vi "Init UART.vi"(6 "Term Char":string, 8 "error in (no error)":errorcluster, 9 "Baud":u32=115200, 10 "UART In":T1=-1, 11 "Session in":refnum<class "Session.lvclass">) -> (0 "error out":errorcluster, 3 "Session out":refnum<class "Session.lvclass">)   [LabVIEW 2020, in "CTI.lvlib" / "Session.lvclass"]
uses:
  Session.lvclass
  Session.lvclass/Session.ctl
  UART/UART.lvclass
  DeviceComms/DeviceComms.lvclass
  UART Number.ctl
  CTI.lvlib
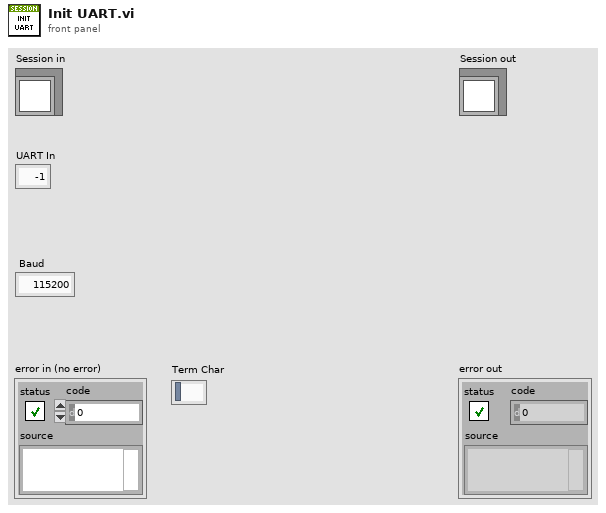
[diagram p1: front panel]
types:
  T1 = typedef "CTI.lvlib/UART Number.ctl" = i8
  T2 = typedef "CTI.lvlib/GPIO Number.ctl" = i8
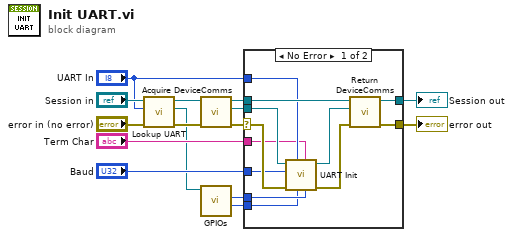
[diagram p0: block diagram]
diagram:
  n1 = call "Lookup UART.vi"("error in (no error)"="error in (no error)", "UART #"="UART In", "Session in"="Session in") -> ("error out"=w5:errorcluster, "UART"=w1:refnum<class "UART.lvclass">, "Session out"=w3:refnum<class "Session.lvclass">)  [unwired: 6 in]
  n2 = call "Acquire DeviceComms.vi"("error in (no error)"=w5, "Session in"=w3) -> ("error out"=w6:errorcluster, "DeviceComms"=w11:refnum<class "DeviceComms.lvclass">, "Session out"=w13:refnum<class "Session.lvclass">)  [unwired: 7 in]
  n3 = call "GPIOs.vi"("UART in"=w1) -> ("RX GPIO"=w7:T2, "TX GPIO"=w8:T2)  [unwired: 7 in, 2 out]
  n4 = case shown="No Error" w6 {
    selector: w6 -> [w27 w29]
    tunnel: [w26 w29] -> w14
    tunnel: w13 -> [w25 w28]
    tunnel: [w24 w28] -> w12
    tunnel: w11 -> [w23 _]
    tunnel: "UART In" -> [w22 _]
    tunnel: "Term Char" -> [w21 _]
    tunnel: "Baud" -> [w20 _]
    tunnel: w8 -> [w19 _]
    tunnel: w7 -> [w18 _]
    frame No Error {
      n5 = call-dynamic "UART Init.vi"("TX GPIO"=w19, "Term Char (None)"=w21, "RX GPIO"=w18, "UART #"=w22, "error in (no error)"=w27, "Baud"=w20, "DeviceComms in"=w23) -> ("error out"=w16:errorcluster, "DeviceComms out"=w17:refnum<class "DeviceComms.lvclass">)  [unwired: 3 in]
      n6 = call "Return DeviceComms.vi"("error in (no error)"=w16, "DeviceComms"=w17, "Session in"=w25) -> ("error out"=w26:errorcluster, "Session out"=w24:refnum<class "Session.lvclass">)  [unwired: 7 in]
    }
    frame Error {
    }
  }
  "error out" <- w14
  "Session out" <- w12
